vi "interakcja_z_plansza.vi"(4 "Controls[] 4":refnum<vi>[](array[refnum]), 6 "Controls[] 6":refnum<vi>[](array[refnum]), 7 "Controls[] 3":refnum<vi>[](array[refnum]), 9 "Controls[]":refnum<vi>[](array[refnum]), 10 "Controls[] 2":refnum<vi>[](array[refnum]), 11 "Controls[] 5":refnum<vi>[](array[refnum])) -> ()   [LabVIEW 2016]
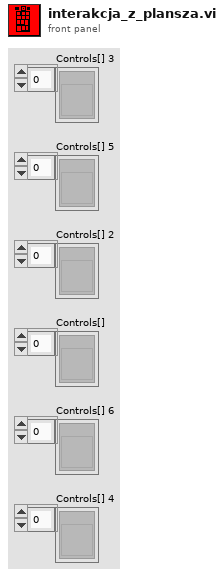
[diagram p1: front panel]
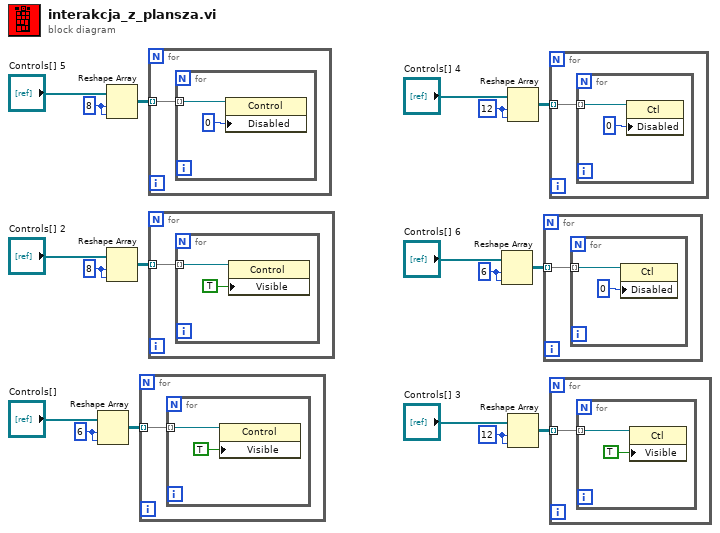
[diagram p0: block diagram]
diagram:
  w11 = 12 ("dimension size")
  w14 = 8 ("dimension size")
  w17 = 6 ("dimension size")
  w8 = 12 ("dimension size")
  w5 = 8 ("dimension size")
  w2 = 6 ("dimension size")
  n1 = Reshape Array("Controls[]", w17, w17) -> (w16:refnum<vi>[][])
  n2 = Reshape Array("Controls[] 5", w5, w5) -> (w4:refnum<vi>[][])
  n3 = Reshape Array("Controls[] 2", w14, w14) -> (w15:refnum<vi>[][])
  n4 = for {
    tunnel: w16 -> [w19] mode=indexing
    n5 = for {
      tunnel: w19 -> [w21] mode=indexing
      n6 = property class="Control"(reference=w21, "Visible"=TRUE) -> ()  [unwired: 1 in, 2 out]
    }
  }
  n7 = for {
    tunnel: w4 -> [w22] mode=indexing
    n8 = for {
      tunnel: w22 -> [w24] mode=indexing
      n9 = property class="Control"(reference=w24, "Disabled"=u8 0) -> ()  [unwired: 1 in, 2 out]
    }
  }
  n10 = for {
    tunnel: w15 -> [w25] mode=indexing
    n11 = for {
      tunnel: w25 -> [w27] mode=indexing
      n12 = property class="Control"(reference=w27, "Visible"=TRUE) -> ()  [unwired: 1 in, 2 out]
    }
  }
  n13 = Reshape Array("Controls[] 6", w2, w2) -> (w3:refnum<vi>[][])
  n14 = Reshape Array("Controls[] 4", w8, w8) -> (w7:refnum<vi>[][])
  n15 = Reshape Array("Controls[] 3", w11, w11) -> (w12:refnum<vi>[][])
  n16 = for {
    tunnel: w3 -> [w28] mode=indexing
    n17 = for {
      tunnel: w28 -> [w30] mode=indexing
      n18 = property class="Ctl"(reference=w30, "Disabled"=u8 0) -> ()  [unwired: 1 in, 2 out]
    }
  }
  n19 = for {
    tunnel: w7 -> [w31] mode=indexing
    n20 = for {
      tunnel: w31 -> [w33] mode=indexing
      n21 = property class="Ctl"(reference=w33, "Disabled"=u8 0) -> ()  [unwired: 1 in, 2 out]
    }
  }
  n22 = for {
    tunnel: w12 -> [w34] mode=indexing
    n23 = for {
      tunnel: w34 -> [w36] mode=indexing
      n24 = property class="Ctl"(reference=w36, "Visible"=TRUE) -> ()  [unwired: 1 in, 2 out]
    }
  }
